vi "EJERCICIO LAZO FOR.vi"() -> ()   [LabVIEW 2020]
panel:
  out "number (0 to 10)":dbl
  out "ITERACIONES":i32
  in  "Numeric":i32
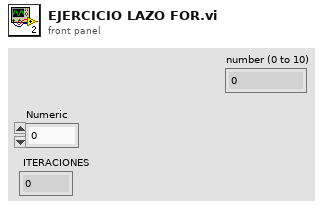
[diagram p1: front panel]
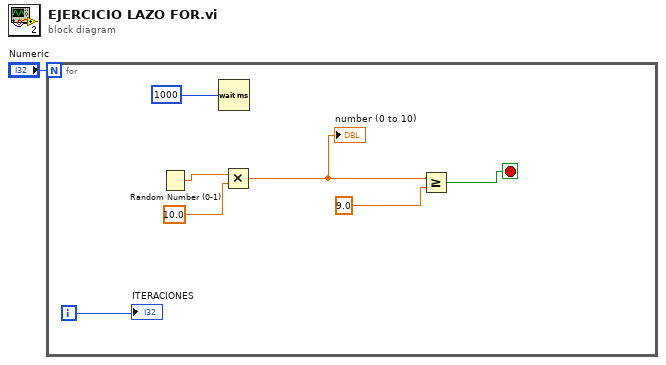
[diagram p0: block diagram]
diagram:
  n1 = for {
    N: "Numeric" -> [_]
    i -> [w3]
    stop <- w2 stop-if-true
    n2 = Random Number (0-1)() -> (number: 0 to 1=w8:dbl)
    n3 = Wait (ms)(milliseconds to wait=u32 1000 ("millisecond timer value")) -> ()  [unwired: 1 out]
    n4 = Multiply(x=w8, y=10.0 ("number (0 to 1)")) -> (x*y=w4:dbl)
    "number (0 to 10)" <- w4
    n5 = Greater Or Equal?(x=w4, y=9.0) -> (x >= y?=w2:bool)
    "ITERACIONES" <- w3
  }
